vi "test json to variant var.vi"(8 "error in (no error)":errorcluster) -> (0 "error out":errorcluster)   [LabVIEW 2019, in "labview_json_tests.lvlib"]
uses:
  labview_json_tests.lvlib
  lib/Element.ctl
  lib/Element Type.ctl
  lib/labview_json.lvlib
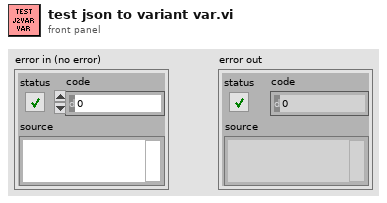
[diagram p1: front panel]
types:
  T1 = typedef "labview_json.lvlib/Element.ctl" = cluster{"Key":string, "Type":T2, "Value":variant}
  T2 = typedef "labview_json.lvlib/Element Type.ctl" = enum8{"NULL", "OBJECT", "ARRAY", "BOOL", "INT", "UINT", "FLOAT", "STRING"}
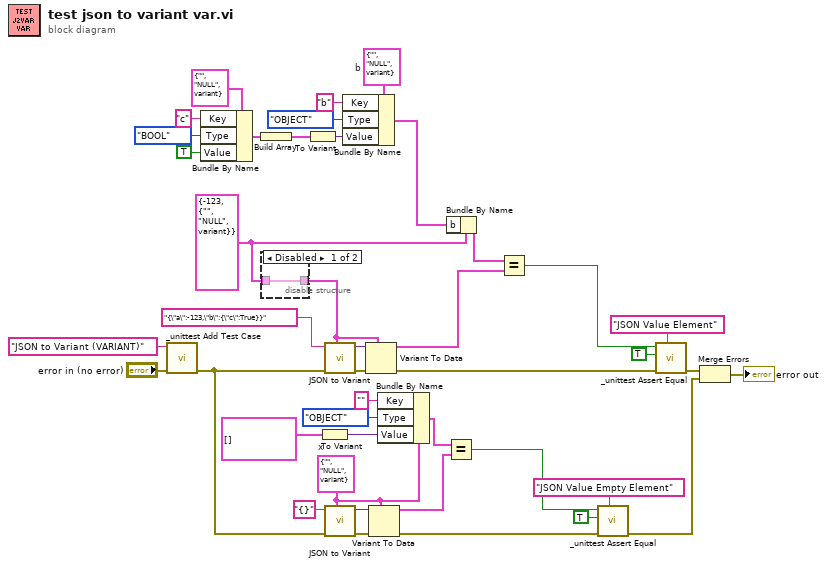
[diagram p0: block diagram]
diagram:
  w24 = T1 {"Key"="", "Type"=enum."NULL", "Value"=variant}  # b
  w9 = T1 {"Key"="", "Type"=enum."NULL", "Value"=variant}  # x
  w25 = cluster{"a":i32, "b":T1} {"a"=-123, "b"={"Key"="", "Type"=enum."NULL", "Value"=variant}} ("Cluster")
  n1 = call "_unittest Add Test Case.vi"("error in (no error)"="error in (no error)", "Test Case"="JSON to Variant (VARIANT)") -> ("error out"=w37:errorcluster)  [unwired: 9 in]
  n2 = Bundle By Name(cluster=T1 {"Key"="", "Type"=enum."NULL", "Value"=variant}, "Key"="c", "Type"=Element_Type."BOOL", "Value"=TRUE) -> (w19:T1)
  n3 = Build Array(w19) -> (w18:T1[])
  n4 = disable-structure shown="Disabled" {
    disable-tunnel: [w43 _] -> w28
    disable-tunnel: w25 -> [w43 _]
    frame Disabled {
    }
    frame Enabled {
    }
  }
  n5 = To Variant(anything=w18) -> (Variant=w14:variant)
  n6 = To Variant(anything=T1[] [] ("appended array")) -> (Variant=w1:variant)
  n7 = call "JSON to Variant.vi"("Variant Type"=w28, "error in (no error)"=w37, "JSON"="{\"a\":-123,\"b\":{\"c\":True}}") -> ("error out"=w26:errorcluster, "Variant out"=w27:variant)  [unwired: 7 in]
  n8 = call "JSON to Variant.vi"("Variant Type"=w9, "error in (no error)"=w37, "JSON"="{}") -> ("error out"=w38:errorcluster, "Variant out"=w33:variant)  [unwired: 7 in]
  n9 = Bundle By Name(cluster=w24, "Key"="b" ("b.Key"), "Type"=Element_Type."OBJECT" ("b.Type"), "Value"=w14) -> (w23:T1)
  n10 = Variant To Data(error in=w26, type=w28, Variant=w27) -> (data=w12:cluster{"a":i32, "b":T1}, error out=w35:errorcluster)
  n11 = Variant To Data(error in=w38, type=w9, Variant=w33) -> (data=w5:T1, error out=w34:errorcluster)
  n12 = Bundle By Name(cluster=w9, "Key"="", "Type"=Element_Type."OBJECT", "Value"=w1) -> (w6:T1)
  n13 = Equal?(x=w6, y=w5) -> (x = y?=w4:bool)
  n14 = Bundle By Name(cluster=w25, "b"=w23) -> (w13:cluster{"a":i32, "b":T1})
  n15 = Equal?(x=w13, y=w12) -> (x = y?=w11:bool)
  n16 = call "_unittest Assert Equal.vi"("Message"="JSON Value Empty Element", "error in (no error)"=w34, "Expected Value"=TRUE, "Actual Value"=w4) -> ("error out"=w36:errorcluster)  [unwired: 7 in]
  n17 = call "_unittest Assert Equal.vi"("Message"="JSON Value Element", "error in (no error)"=w35, "Expected Value"=TRUE, "Actual Value"=w11) -> ("error out"=w40:errorcluster)  [unwired: 7 in]
  n18 = Merge Errors(w40, w36) -> (→"error out":errorcluster)
